vi "WriteHeader.vi"(0 "Buffers in":T1={"Channels"=[], "PosttriggerBuffer"=refnum, "PretriggerBuffer"=refnum, "BlockSizePerChannel"=0, " logging semaphore"=refnum, "Log refnum"=refnum, "snapshotBuffer"=refnum, "logDirectory"=path "", "logPrefix"="", "decimation factor"=1, "max files"=0, "SampleRate"=0.0}, 1 "LogMetaData":cluster{"Property":string, "value":variant}[](array[cluster]), 11 "error in (no error)":errorcluster) -> (4 "Buffers out":T1={"Channels"=[], "PosttriggerBuffer"=refnum, "PretriggerBuffer"=refnum, "BlockSizePerChannel"=0, " logging semaphore"=refnum, "Log refnum"=refnum, "snapshotBuffer"=refnum, "logDirectory"=path "", "logPrefix"="", "decimation factor"=1, "max files"=0, "SampleRate"=0.0}, 8 "numOfChannels":i32, 15 "error out":errorcluster)   [LabVIEW 2015, in "BufferLogging.lvlib"]
uses:
  BufferLogging.lvlib
  Buffers.ctl
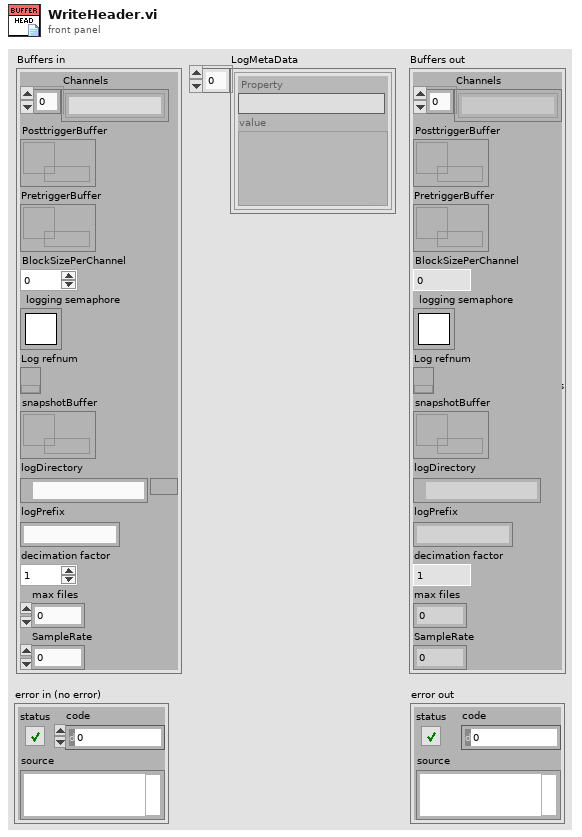
[diagram p1: front panel]
types:
  T1 = typedef "BufferLogging.lvlib/Buffers.ctl" = cluster{"Channels":string[], "PosttriggerBuffer":refnum<queue>, "PretriggerBuffer":refnum<queue>, "BlockSizePerChannel":i32, " logging semaphore":T2, "Log refnum":refnum<k34>, "snapshotBuffer":refnum<data-value>, "logDirectory":path, "logPrefix":string, "decimation factor":i32, "max files":i32, "SampleRate":dbl}
  T2 = typedef "Semaphore RefNum" = refnum<k1>
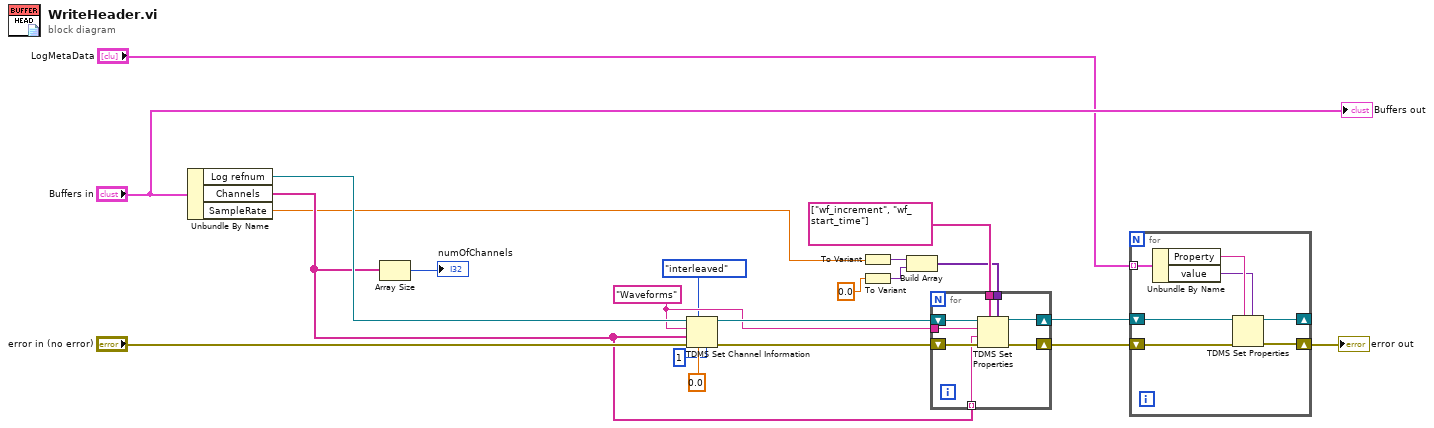
[diagram p0: block diagram]
diagram:
  w15 = "Waveforms" ("group name (Untitled)")
  n1 = Unbundle By Name("Buffers in") -> ("Log refnum"=w19:refnum<k34>, "Channels"=w2:string[], "SampleRate"=w1:dbl)
  n2 = Array Size(array=w2) -> (size(s)=→"numOfChannels":i32)
  n3 = TDMS Set Channel Information(4:u32 1 ("samples per channel"), 6:sgl 0.0, 7:enum16{"non-interleaved", "interleaved"}."interleaved" ("data layout (0:non-interleaved)"), 8:"error in (no error)", 9:w2, 10:w15, 11:w19) -> (0:w17:errorcluster, 3:w16:refnum<k34>)
  n4 = To Variant(anything=w1) -> (Variant=w9:variant)
  n5 = To Variant(anything=0.0) -> (Variant=w8:variant)
  n6 = Build Array(w9, w8) -> (w7:variant[])
  n7 = for {
    tunnel: w15 -> [w26]
    tunnel: string[] ["wf_increment", "wf_start_time"] ("property names") -> [w25]
    tunnel: w7 -> [w24]
    shift-right: [w27] -> w6
    shift-left: w17 -> [w29]
    tunnel: w2 -> [w23] mode=indexing
    shift-right: [w22] -> w4
    shift-left: w16 -> [w28]
    n8 = TDMS Set Properties(5:w24, 7:w25, 8:w29, 9:w23, 10:w26, 11:w28) -> (0:w27:errorcluster, 3:w22:refnum<k34>)  [unwired: 2 out]
  }
  n9 = for {
    shift-right: [w35] -> w5
    shift-left: w6 -> [w36]
    shift-right: [w34] -> _
    shift-left: w4 -> [w32]
    tunnel: "LogMetaData" -> [w33] mode=indexing
    n10 = Unbundle By Name(w33) -> ("Property"=w31:string, "value"=w30:variant)
    n11 = TDMS Set Properties(5:w30, 7:w31, 8:w36, 11:w32) -> (0:w35:errorcluster, 3:w34:refnum<k34>)  [unwired: 2 in, 2 out]
  }
  "error out" <- w5
  "Buffers out" <- "Buffers in"
